vi "hmp4000 Configure Voltage Value.vi"(8 "error in (no error)":errorcluster, 9 "Voltage (0.0)":dbl format="%.3f", 11 "VISA resource name":refnum<visa-resource-name>) -> (0 "error out":errorcluster, 3 "VISA resource name out":refnum<visa-resource-name>)   [LabVIEW 2022 SP3]
doc: "This VI adjusts the output voltage level.\n\nAttribute:\nHMP4000_ATTR_OUTPUT_VOLTAGE_LEVEL\n\nRemote-control command:\nSOURce:VOLTage:LEVel:AMPLitude"
uses:
  Instance           1 39Saved   hmp4000 Configure Voltage Value .vi
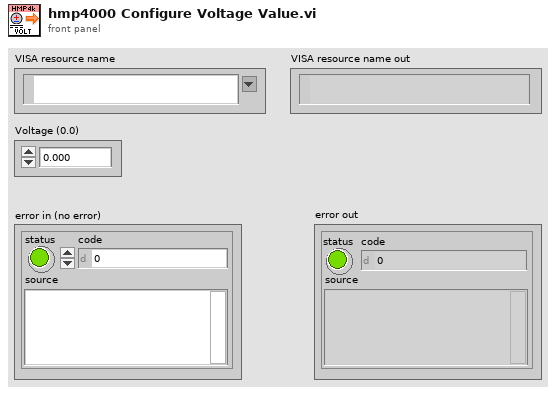
[diagram p1: front panel]
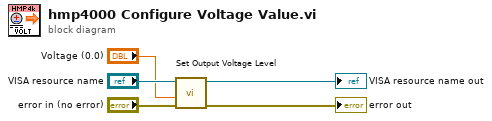
[diagram p0: block diagram]
diagram:
  n1 = call "Set Output Voltage Level"("error in (no error)"="error in (no error)", "Output Voltage Level (0.0)"="Voltage (0.0)", "instrument handle"="VISA resource name") -> ("error out"=→"error out":errorcluster, "instrument handle out"=→"VISA resource name out":refnum<visa-resource-name>)  [unwired: 7 in]
